vi "TRAFFIC LIGHT.vi"() -> ()   [LabVIEW 2019]
panel:
  in  "?":bool
  out "GREEN":bool
  out "YELLOW":bool
  out "RED":bool
  out "TIMER":dbl
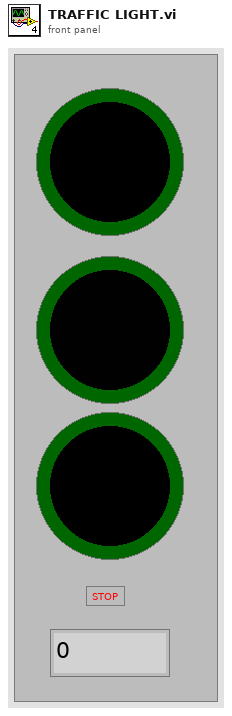
[diagram p1: front panel]
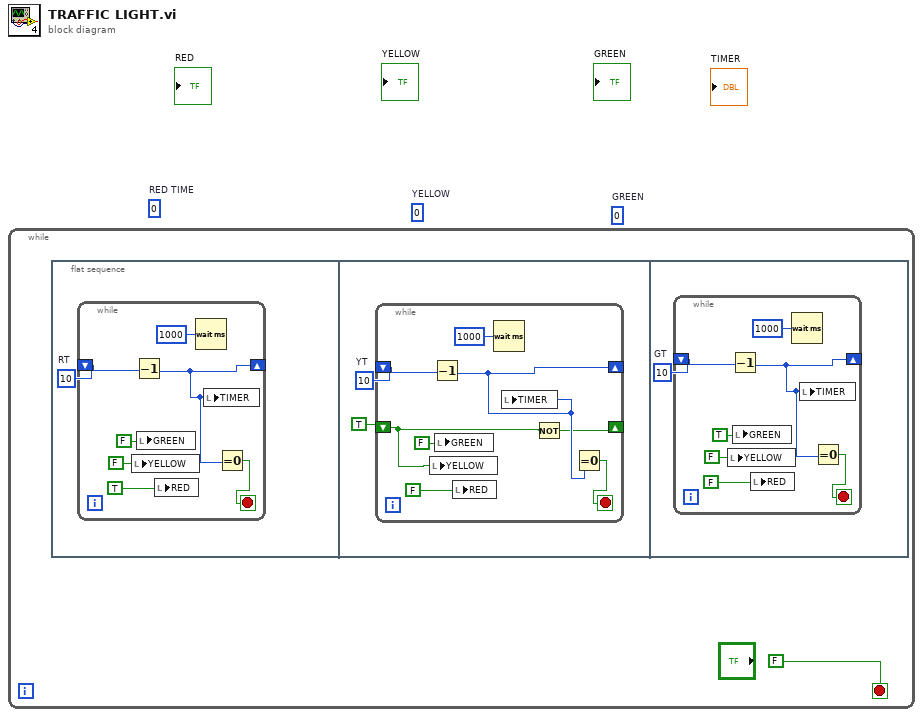
[diagram p0: block diagram]
diagram:
  (unwired) 0  # GREEN
  (unwired) 0  # RED TIME
  (unwired) 0  # YELLOW
  n1 = while {
    stop <- FALSE stop-if-true
    n2 = flat-sequence {
      frame #0 {
        w2 = 10  # RT
        n3 = while {
          shift-right: [w4] -> _
          shift-left: w2 -> [w6]
          stop <- w5 stop-if-true
          n4 = local write "YELLOW"(FALSE) -> ()
          n5 = Decrement(x=w6) -> (x-1=w4:i32)
          n6 = local write "GREEN"(FALSE) -> ()
          n7 = local write "RED"(TRUE) -> ()
          n8 = Wait (ms)(milliseconds to wait=u32 1000) -> ()  [unwired: 1 out]
          n9 = local write "TIMER"(w4) -> ()
          n10 = Equal To 0?(x=w4) -> (x = 0?=w5:bool)
        }
      }
      frame #1 {
        w11 = 10  # YT
        n11 = while {
          shift-right: [w15] -> _
          shift-left: w11 -> [w17]
          shift-right: [w12] -> _
          shift-left: TRUE -> [w13]
          stop <- w16 stop-if-true
          n12 = local write "YELLOW"(w13) -> ()
          n13 = Decrement(x=w17) -> (x-1=w15:i32)
          n14 = local write "GREEN"(FALSE) -> ()
          n15 = local write "RED"(FALSE) -> ()
          n16 = Wait (ms)(milliseconds to wait=u32 1000) -> ()  [unwired: 1 out]
          n17 = local write "TIMER"(w15) -> ()
          n18 = Not(x=w13) -> (.not. x?=w12:bool)
          n19 = Equal To 0?(x=w15) -> (x = 0?=w16:bool)
        }
      }
      frame #2 {
        w20 = 10  # GT
        n20 = while {
          shift-right: [w22] -> _
          shift-left: w20 -> [w24]
          stop <- w23 stop-if-true
          n21 = local write "YELLOW"(FALSE) -> ()
          n22 = Decrement(x=w24) -> (x-1=w22:i32)
          n23 = local write "GREEN"(TRUE) -> ()
          n24 = local write "RED"(FALSE) -> ()
          n25 = Wait (ms)(milliseconds to wait=u32 1000) -> ()  [unwired: 1 out]
          n26 = local write "TIMER"(w22) -> ()
          n27 = Equal To 0?(x=w22) -> (x = 0?=w23:bool)
        }
      }
    }
  }
